vi "Setting-CT.vi"(8 "error in (no error)":errorcluster, 10 "number":i32, 11 "VISA resource name":refnum<visa-resource-name>) -> (0 "error out":errorcluster, 3 "VISA resource name 2":refnum<visa-resource-name>)   [LabVIEW 2017]
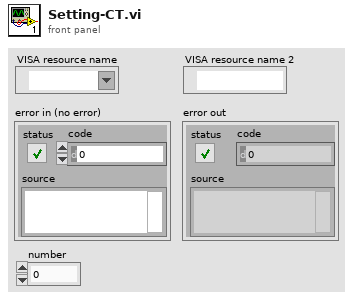
[diagram p1: front panel]
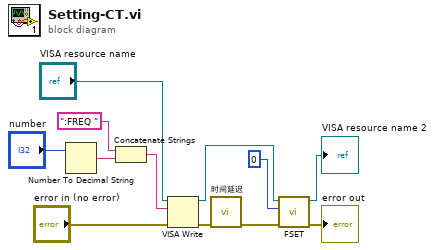
[diagram p0: block diagram]
diagram:
  n1 = Number To Decimal String(number="number") -> (decimal integer string=w11:string)  [unwired: 1 in]
  n2 = Concatenate Strings(":FREQ " ("字符串"), w11) -> (w10:string)
  n3 = VISA Write(VISA resource name="VISA resource name", write buffer=w10, error in (no error)="error in (no error)") -> (VISA resource name out=w2:refnum<visa-resource-name>, error out=w5:errorcluster)  [unwired: 1 out]
  n4 = call "时间延迟"("error in (no error)"=w5) -> ("error out"=w4:errorcluster)  [unwired: 10 in]
  n5 = call "FSET.vi"("error in (no error)"=w4, "Function (0: Cp-D)"=0, "VISA resource name"=w2) -> ("error out"=→"error out":errorcluster, "VISA resource name out"=→"VISA resource name 2":refnum<visa-resource-name>)  [unwired: 7 in]
